vi "CRYGraph View Socket Client.vi"(8 "sOption":string, 9 "nData":i32, 10 "sData":string, 11 "sAction":string) -> (0 "bResult Out":bool, 1 "sData Out":string, 2 "Variant Out":variant[](array[variant]), 3 "pVI Out":refnum<vi>)   [LabVIEW 2013]
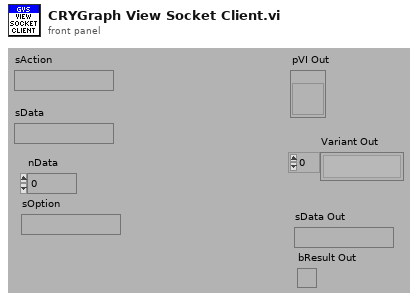
[diagram p1: front panel]
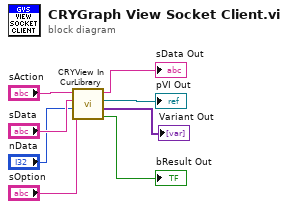
[diagram p0: block diagram]
diagram:
  n1 = call "CRYView In CurLibrary.vi"("sOption"="sOption", "nData"="nData", "sData"="sData", "sAction"="sAction") -> ("bResult"=→"bResult Out":bool, "pRefList_Out"=→"Variant Out":variant[], "pVIRef_Out"=→"pVI Out":refnum<vi>, "SData_Out"=→"sData Out":string)  [unwired: 4 in]
